vi "Cache.Result.ComponentAdd.vi"(6 "Time (now)":timestamp, 7 "Idx":i32, 8 "error in (no error)":errorcluster, 10 "ProdComp":T1) -> (0 "error out":errorcluster)   [LabVIEW 2016]
uses:
  Cache.ProductComponent.Data.ctl
  Tools/Translator/Translator.Message.ctl
  Tools/EventLog/EventLog.EventSource.ctl
  Tools/EventLog/EventLog.New(array).vi
  Global/ApplicationGlobal.vi
  Tools/EventLog/EventLog.Buffer.vi
  Tools/EventLog/EventLog.File.ReadWrite.vi
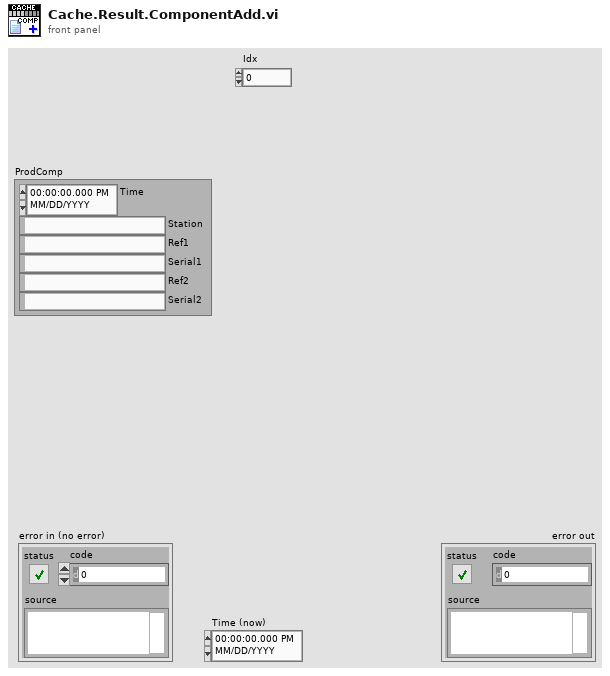
[diagram p1: front panel]
types:
  T1 = typedef "Cache.ProductComponent.Data.ctl" = cluster{"Time":timestamp, "Station":string, "Ref1":string, "Serial1":string, "Ref2":string, "Serial2":string}
  T2 = typedef "EventLog.EventSource.ctl" = enum16{"All", "Gui", "PLC1", "PLC2", "PLC3", "DB", "DB01", "DB02", "DB03", "DB04", "DB05", "DB06", "DB07", "DB08", "DB09", "DB10", "DB11", "DB12", "DB13", "DB14", "DB15", "DB16"}
  T3 = typedef "Translator.Message.ctl" = enum16{"-", "Event confirmed", "Log out", "Log in", "Shutdown", "Cancel", "Start", "Continue", "Stop", "On", "Off", "OK", "NOK", "NOK %s", "This", "Prev", "Home", "Work", "In progress...", "Missing", "Empty", "Hardware failure", "Initial", "Error %d >> %s", "Error %d >> %s >> %s", "Starting %s", "Quitting %s", "Configured", "Initializing", "Quitting", "Loading", "Running %s", "Stopped", "Summary", "Do you want to continue?", "Do you want to exit?", "Log out?", "System", "All", "IDLE", "Translating...%s", "Not found", "Alarm %s", "Run", "Skip", "Abort", "Repeat", "Please wait...", "Database disconnected", "Login to database successful", "Login to database failed: %d; %s", "Get process step data for %s", "Changeover off", "Changeover into %s", "Product %s | %s found in cache with status %d at previous station", "Product %s | %s found in database with status %d at previous station", "Product %s | %s not found in cache at previous station", "Product %s | %s not found in database at previous station", "Product %s | %s found in cache with status %d at this station (%d repetion)", "Product %s | %s found in database with status %d at this station (%d repetition)", "Product %s | %s not found in cache at this station", "Product %s | %s not found in database at this station", "Product %s | %s found in cache for component %s | %s", "Product %s | %s found in database for component %s | %s", "Product not found in cache for component %s | %s", "Product not found in database for component %s | %s", "Product %s | %s connected with component %s | %s (cache)", "Product %s | %s connected with component %s | %s (database)", "New data for %s | %s (cache)", "New data for %s | %s (database)", "Msg %d >> %s", "PLC LifeBit Failure", "Reconnecting DB", "Reconnecting PLC"}
  T4 = enum16{"open", "open or create", "create or replace", "create", "open (read-only)"}
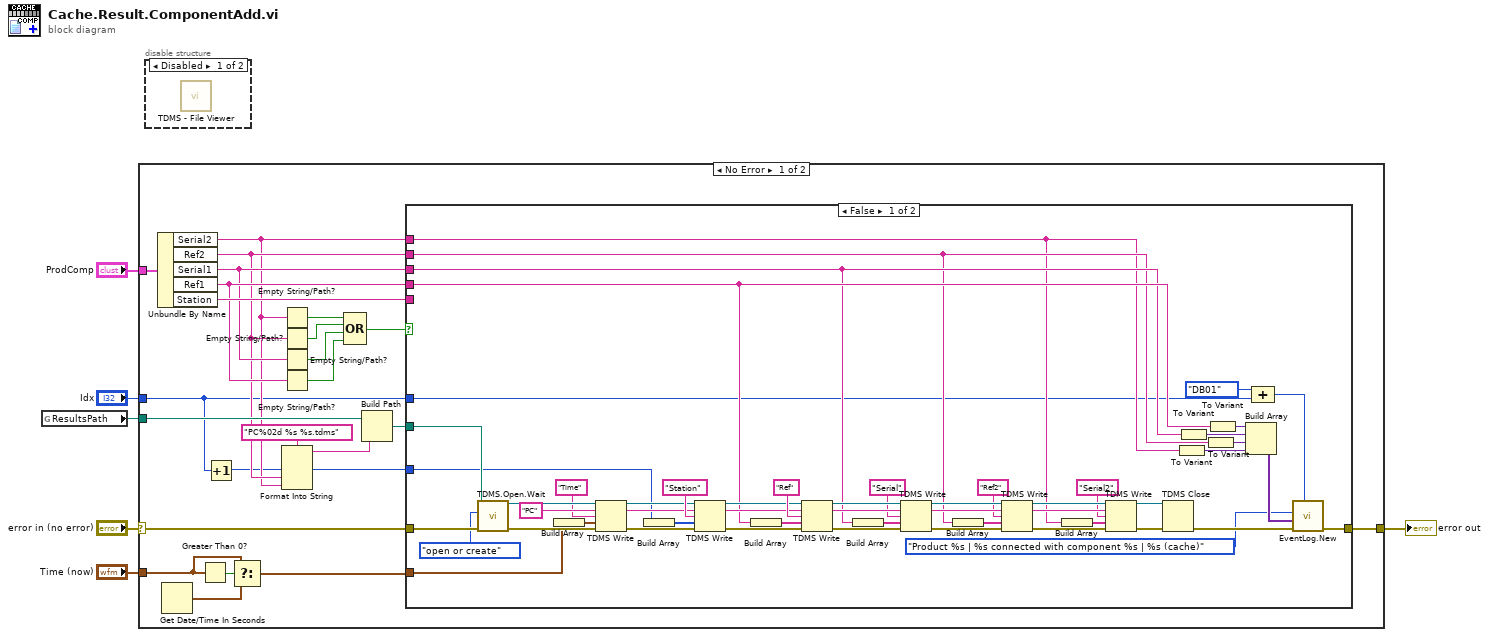
[diagram p0: block diagram]
diagram:
  n1 = global read "ApplicationGlobal.vi" "ResultsPath"() -> (w3:path)
  n2 = case shown="No Error" "error in (no error)" {
    selector: "error in (no error)" -> [w28 w83]
    tunnel: [w29 w83] -> w6
    tunnel: "ProdComp" -> [w27 _]
    tunnel: w3 -> [w21 _]
    tunnel: "Idx" -> [w8 _]
    tunnel: "Time (now)" -> [w12 _]
    frame No Error {
      n3 = Unbundle By Name(w27) -> ("Serial2"=w10:string, "Ref2"=w11:string, "Serial1"=w15:string, "Ref1"=w16:string, "Station"=w19:string)
      n4 = Get Date/Time In Seconds() -> (seconds since 1Jan1904=w13:timestamp)
      n5 = Greater Than 0?(x=w12) -> (x > 0?=w14:bool)
      n6 = Increment(x=w8) -> (x+1=w7:i32)
      n7 = Select(t=w12, s=w14, f=w13) -> (s? t:f=w9:timestamp)
      n8 = Empty String/Path?(string/path=w10) -> (empty?=w26:bool)
      n9 = Empty String/Path?(string/path=w11) -> (empty?=w25:bool)
      n10 = Empty String/Path?(string/path=w15) -> (empty?=w24:bool)
      n11 = Empty String/Path?(string/path=w16) -> (empty?=w23:bool)
      n12 = Format Into String(format string="PC%02d %s %s.tdms" ("pattern"), w7, w11, w10) -> (resulting string=w17:string)  [unwired: 2 in, 1 out]
      n13 = Compound Arithmetic op=OR(w26, w25, w24, w23) -> (w22:bool)
      n14 = Build Path(base path=w21, name or relative path=w17) -> (appended path=w20:path)
      n15 = case shown="False" w22 {
        tunnel: [w51 w82] -> w29
        tunnel: w28 -> [w81 w82]
        tunnel: w11 -> [w48 _]
        tunnel: w10 -> [w47 _]
        tunnel: w15 -> [w49 _]
        tunnel: w16 -> [w50 _]
        tunnel: w20 -> [w60 _]
        tunnel: w19 -> [_ _]
        tunnel: w8 -> [w40 _]
        tunnel: w9 -> [w30 _]
        tunnel: w7 -> [w31 _]
        frame False {
          n16 = call "TDMS.Open.Wait.vi"("error in (no error)"=w81, "operation (open read-only)"=T4."open or create" ("operation (0:open)"), "file path"=w60) -> ("error out"=w37:errorcluster, "tdms file out"=w38:refnum<k34>)  [unwired: 7 in]
          n17 = Build Array(w30) -> (w33:timestamp[])
          n18 = TDMS Write(0:w38, 5:"PC" ("date/time string"), 7:"Time", 9:w33, 11:w37) -> (4:w36:refnum<k34>, 6:w35:string, 15:w34:errorcluster)  [unwired: 1 in, 1 out]
          n19 = Build Array(w31) -> (w59:i32[])
          n20 = TDMS Write(0:w36, 5:w35, 7:"Station", 9:w59, 11:w34) -> (4:w56:refnum<k34>, 6:w55:string, 15:w57:errorcluster)  [unwired: 1 in, 1 out]
          n21 = Build Array(w50) -> (w80:string[])
          n22 = TDMS Write(0:w56, 5:w55, 7:"Ref", 9:w80, 11:w57) -> (4:w78:refnum<k34>, 6:w77:string, 15:w79:errorcluster)  [unwired: 1 in, 1 out]
          n23 = Build Array(w49) -> (w76:string[])
          n24 = TDMS Write(0:w78, 5:w77, 7:"Serial", 9:w76, 11:w79) -> (4:w72:refnum<k34>, 6:w73:string, 15:w74:errorcluster)  [unwired: 1 in, 1 out]
          n25 = Build Array(w48) -> (w75:string[])
          n26 = TDMS Write(0:w72, 5:w73, 7:"Ref2", 9:w75, 11:w74) -> (4:w66:refnum<k34>, 6:w65:string, 15:w69:errorcluster)  [unwired: 1 in, 1 out]
          n27 = Build Array(w47) -> (w63:string[])
          n28 = TDMS Write(0:w66, 5:w65, 7:"Serial2", 9:w63, 11:w69) -> (4:w68:refnum<k34>, 15:w67:errorcluster)  [unwired: 1 in, 2 out]
          n29 = TDMS Close(8:w67, 11:w68) -> (0:w52:errorcluster)  [unwired: 1 out]
          n30 = To Variant(anything=w47) -> (Variant=w45:variant)
          n31 = To Variant(anything=w49) -> (Variant=w54:variant)
          n32 = To Variant(anything=w48) -> (Variant=w46:variant)
          n33 = To Variant(anything=w50) -> (Variant=w53:variant)
          n34 = Build Array(w53, w54, w46, w45) -> (w44:variant[])
          n35 = Compound Arithmetic op=ADD(EventLog.EventSource."DB01" ("Source (All)"), w40) -> (w41:i32)
          n36 = call-poly "EventLog.New.vi"("Source (All)"=w41, "error in (no error)"=w52, "Arguments"=w44, "Message (-)"=Translator.Message."Product %s | %s connected with component %s | %s (cache)") -> ("error out"=w51:errorcluster)  [unwired: 6 in, 1 out]
        }
        frame True {
        }
      }
    }
    frame Error {
    }
  }
  "error out" <- w6
  n37 = disable-structure shown="Disabled" {
    frame Disabled {
      n38 = call <vilib>:"TDMS - File Viewer.vi"() -> ()  [unwired: 6 in, 2 out]
    }
    frame Enabled {
    }
  }
